vi "Dialog - list update.vi"(9 "Files to add":string[](array[string]), 11 "Lists":string[](array[string])) -> (1 "selected list":string, 3 "files":string[](array[string]))   [LabVIEW 2022 SP3]
panel:
  in  "update":bool
  in  "Cancel Button":bool
  in  "Existing lists":u16(ring) items=["Currently open....", "Strads"]
  # "Select the list to update"
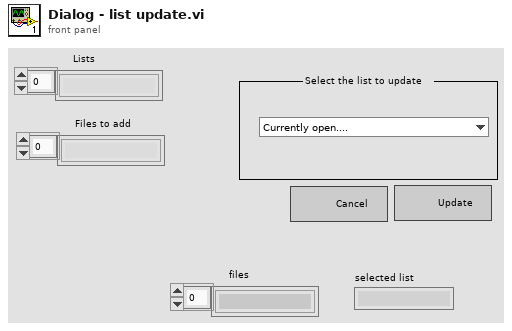
[diagram p1: front panel]
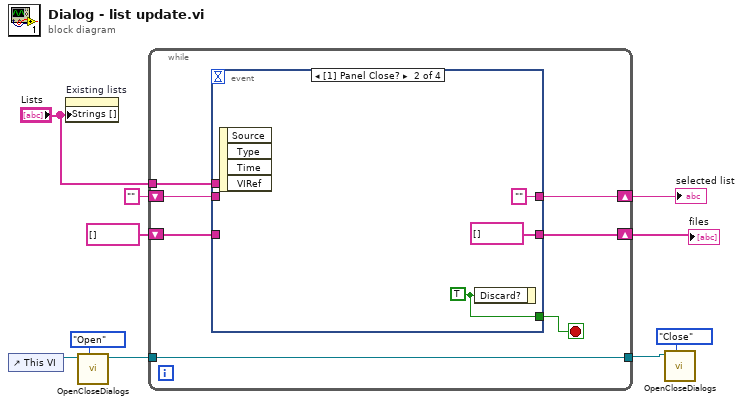
[diagram p0: block diagram]
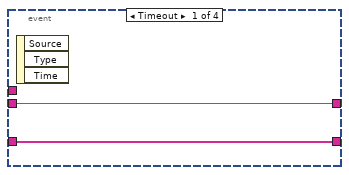
[diagram p2: hidden frame]
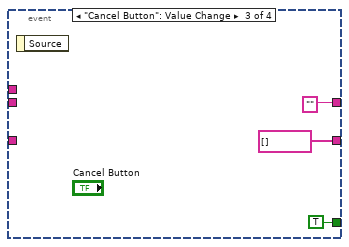
[diagram p3: hidden frame]
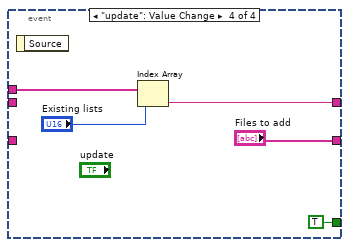
[diagram p4: hidden frame]
diagram:
  n1 = control-ref of="This VI"() -> (w9:refnum<vi>)
  n2 = property on="Existing lists" class="Ring (strict)"("Strings []"="Lists") -> ()  [unwired: 2 in, 2 out]
  n3 = call "OpenCloseDialogs.vi"("Task"=enum16{"Open", "Close"}."Open", "VI in"=w9) -> ("VI out"=w7:refnum<vi>)  [unwired: 8 in, 1 out]
  n4 = while {
    tunnel: [w16] -> w6
    tunnel: w7 -> [w16]
    tunnel: "Lists" -> [w15]
    shift-right: [w14] -> w4
    shift-left: "" ("String") -> [w13]
    shift-right: [w12] -> w2
    shift-left: string[] [] ("Files to add") -> [w11]
    stop <- w17 stop-if-true
    n5 = event shown="[1] Panel Close?" {
      selector: _ -> [_ _ _ _]
      dyn-events: _ -> [_ _ _ _]
      timeout: _ -> [_ _ _ _]
      tunnel: [_ w22 TRUE ("Discard?") TRUE ("Discard?")] -> w17
      tunnel: w15 -> [_ _ _ w29]
      tunnel: [w19 "" ("String") "" ("String") w28] -> w14
      tunnel: w13 -> [w19 _ _ _]
      tunnel: [w18 string[] [] ("Files to add") string[] [] ("Files to add") "Files to add"] -> w12
      tunnel: w11 -> [w18 _ _ _]
      event Timeout {
        n6 = event-data() -> ()  [unwired: 1 in, 3 out]
      }
      event Panel Close? {
        w22 = TRUE ("Discard?")
        n7 = event-data() -> ()  [unwired: 1 in, 4 out]
        n8 = event-data("Discard?"=w22) -> ()  [unwired: 1 in, 1 out]
      }
      event "Cancel Button": Value Change {
        n9 = event-data() -> ()  [unwired: 1 in, 1 out]
      }
      event "update": Value Change {
        n10 = event-data() -> ()  [unwired: 1 in, 1 out]
        n11 = Index Array(array=w29, index="Existing lists") -> (element=w28:string)
      }
    }
  }
  "selected list" <- w4
  "files" <- w2
  n12 = call "OpenCloseDialogs.vi"("Task"=enum16{"Open", "Close"}."Close", "VI in"=w6) -> ()  [unwired: 8 in, 2 out]
